vi "VCC_subVI.vi"(1 "Velocidade Desejada":i16(slide) min=0 max=4500 step=100 scale=0.0..4500.0, 2 "VISA resource name":refnum<visa-resource-name>) -> (0 "Velocidade Real":i16)   [LabVIEW 2019]
uses:
  <vilib>/Instr/_visa.llb/VISA Configure Serial Port (Instr).vi
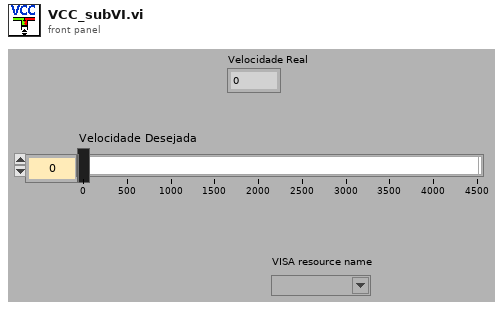
[diagram p1: front panel]
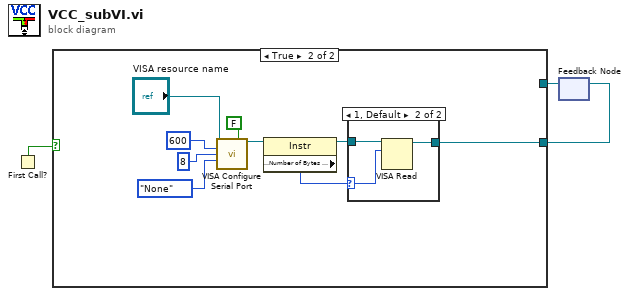
[diagram p0: block diagram]
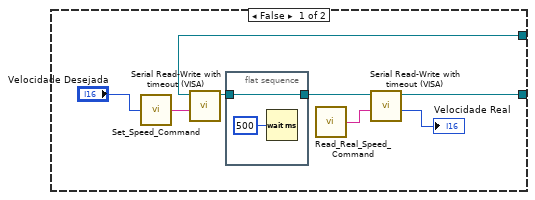
[diagram p2: hidden frame]
diagram:
  n1 = First Call?() -> (First Call?: T/F=w3:bool)
  n2 = feedback #1() -> (w1:refnum<visa-resource-name>)  [unwired: 1 in]
  n3 = case shown="True" w3 {
    tunnel: [w4 w15] -> w2
    tunnel: w1 -> [w5 _]
    frame False {
      n4 = call "Set_Speed_Command.vi"("Speed Control"="Velocidade Desejada") -> ("Speed Control String to send:"=w11:string)
      n5 = call "Serial Read-Write with timeout (VISA).vi"("Write String"=w11, "VISA session"=w5) -> ("VISA session out"=w9:refnum<visa-resource-name>)  [unwired: 2 in, 3 out]
      n6 = flat-sequence {
        tunnel: w9 -> [w13]
        tunnel: [w13] -> w8
        frame #0 {
          n7 = Wait (ms)(milliseconds to wait=u32 500) -> ()  [unwired: 1 out]
        }
      }
      n8 = call "Read_Real_Speed_Command.vi"() -> ("Read Real Speed String to send:"=w10:string)
      n9 = call "Serial Read-Write with timeout (VISA).vi"("Write String"=w10, "VISA session"=w8) -> ("Speed"=→"Velocidade Real":i16, "VISA session out"=w4:refnum<visa-resource-name>)  [unwired: 2 in, 2 out]
    }
    frame True {
      n10 = call-poly "VISA Configure Serial Port"("VISA resource name"="VISA resource name", "Enable Termination\nChar (T)"=FALSE ("Enable Termination\nChar (T)"), "baud rate (9600)"=u32 600, "data bits (8)"=u16 8, "parity (0:none)"=enum16{"None", "Odd", "Even", "Mark", "Space"}."None") -> ("VISA resource name out"=w18:refnum<visa-resource-name>)  [unwired: 9 in, 1 out]
      n11 = property class="Instr"(reference=w18) -> (reference out=w19:refnum<visa-resource-name>, "Serial Settings:Number of Bytes at Serial Port"=w17:u32)  [unwired: 1 in, 1 out]
      n12 = case shown="1, Default" w17 {
        selector: w17 -> [_ w24]
        tunnel: w19 -> [w23 w26]
        tunnel: [w23 w25] -> w15
        frame 0 {
        }
        frame 1, Default {
          n13 = VISA Read(VISA resource name=w26, byte count=w24) -> (VISA resource name out=w25:refnum<visa-resource-name>)  [unwired: 1 in, 3 out]
        }
      }
    }
  }
  n14 = feedback-in #1(w2) -> ()
